vi "IP check.vi"(11 "IP address string":string) -> (2 "Valid?":bool)   [LabVIEW 2021]
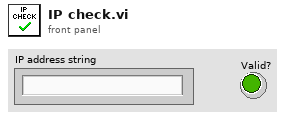
[diagram p1: front panel]
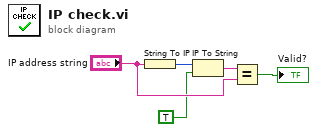
[diagram p0: block diagram]
diagram:
  n1 = String To IP(1:"IP address string") -> (0:w3:u32)
  n2 = IP To String(1:TRUE ("dot notation? (F)"), 2:w3) -> (0:w2:string)
  n3 = Equal?(x=w2, y="IP address string") -> (x = y?=→"Valid?":bool)
